vi "template_Job_Minimal.vi"() -> ()   [LabVIEW 2013]
panel:
  out "error out":errorcluster
  out "stdout":string
  in  "stdin":string
  # "All Controls and Indicators are optional and can be deleted\n\n-- stdin allows to pass in commands into the job\n-- stdout allows to send back a response to the scheduler after execution completes\n-- error output terminal returns the exception code to the scheduler\n-- stdin and stdout are default labels. If they are to be named differently, one must configure the constructor node declaring the Static VI refnum."
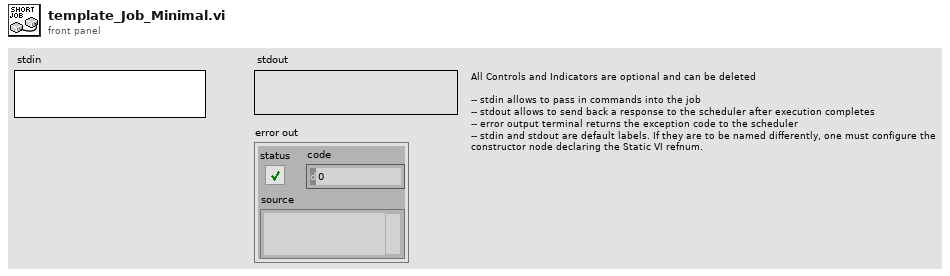
[diagram p1: front panel]
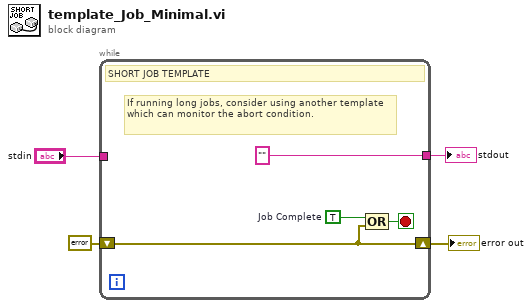
[diagram p0: block diagram]
diagram:
  n1 = while {
    shift-right: [w7] -> w2
    shift-left: errorcluster {"status"=FALSE, "code"=0, "source"=""} ("error out") -> [w7]
    tunnel: "stdin" -> [_]
    tunnel: [""] -> w1
    stop <- w8 stop-if-true
    w6 = TRUE  # Job Complete
    # "If running long jobs, consider using another template which can monitor the abort condition."
    # "SHORT JOB TEMPLATE"
    n2 = Compound Arithmetic op=OR(w6, w7) -> (w8:bool)
  }
  "error out" <- w2
  "stdout" <- w1
